vi "规范分钟时间戳.vi"(11 "字符串":string) -> (3 "result string":string)   [LabVIEW 2016]
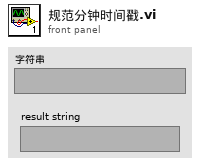
[diagram p1: front panel]
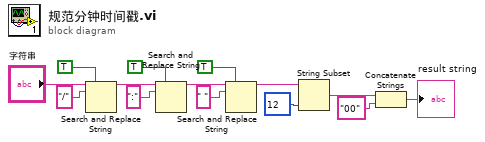
[diagram p0: block diagram]
diagram:
  n1 = Search and Replace String(replace all?=TRUE ("替换全部？(F)"), input string="字符串", search string="/" ("搜索字符串")) -> (result string=w6:string)  [unwired: 5 in, 3 out]
  n2 = Search and Replace String(replace all?=TRUE ("替换全部？(F)"), input string=w6, search string=":" ("搜索字符串")) -> (result string=w5:string)  [unwired: 5 in, 3 out]
  n3 = Search and Replace String(replace all?=TRUE ("替换全部？(F)"), input string=w5, search string=" " ("搜索字符串")) -> (result string=w10:string)  [unwired: 5 in, 3 out]
  n4 = String Subset(string=w10, length (rest)=12 ("长度（剩余）")) -> (substring=w12:string)  [unwired: 1 in]
  n5 = Concatenate Strings(w12, "00" ("字符串")) -> (→"result string":string)
